vi "GetParam.vi"(8 "error in (no error)":errorcluster caption="entrée d'erreur (pas d'erreur)", 11 "V_Measure_Score.lvclass":refnum<class "V_Measure_Score.lvclass">) -> (0 "error out":errorcluster caption="sortie d'erreur", 2 "v_measure_score":cluster{"beta":dbl}={"beta"=1.0}, 3 "V_Measure_Score.lvclass":refnum<class "V_Measure_Score.lvclass">)   [LabVIEW 2020, in "V_Measure_Score.lvclass"]
doc: "Get Parameters"
uses:
  V_Measure_Score.lvclass
  V_Measure_Score.lvclass/V_Measure_Score.ctl
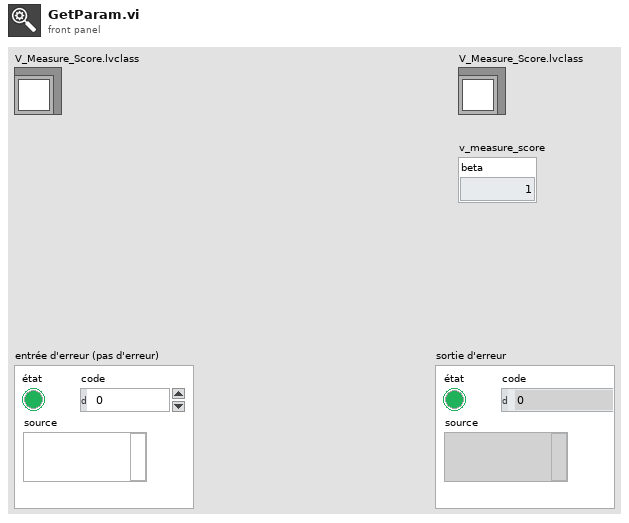
[diagram p1: front panel]
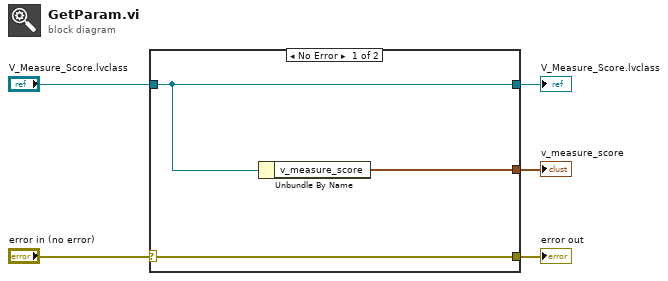
[diagram p0: block diagram]
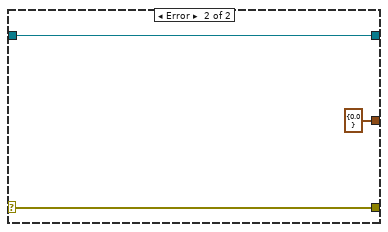
[diagram p2: hidden frame]
diagram:
  n1 = case shown="No Error" "error in (no error)" {
    selector: "error in (no error)" -> [w8 w10]
    tunnel: [w8 w10] -> w4
    tunnel: [w7 w11] -> w2
    tunnel: "V_Measure_Score.lvclass" -> [w7 w11]
    tunnel: [w6 cluster{"beta":dbl} {"beta"=0.0} ("v_measure_score")] -> w1
    frame No Error {
      n2 = Unbundle By Name(w7) -> ("v_measure_score"=w6:cluster{"beta":dbl})
    }
    frame Error {
    }
  }
  "error out" <- w4
  "V_Measure_Score.lvclass" <- w2
  "v_measure_score" <- w1
